vi "Beta Moments.vi"(9 "b":dbl=1.0, 10 "a":dbl=1.0) -> (0 "error":i32, 2 "variance":dbl=0.08333333333333333, 3 "mean":dbl=0.5)   [LabVIEW 2017, in "NI_Gmath.lvlib"]
doc: "Returns the expected mean and variance of the random variate X, where X describes the selected distribution type. You must manually select the polymorphic instance to use."
uses:
  <vilib>/gmath/NI_Gmath.lvlib
  <vilib>/gmath/statdist.llb/st_error_code.ctl
panel:
  # "Beta Moments"
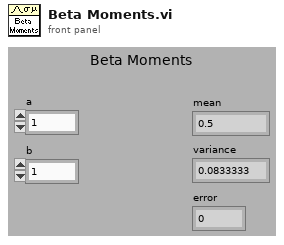
[diagram p1: front panel]
types:
  T1 = typedef "NI_Gmath.lvlib/st_error_code.ctl" = i32
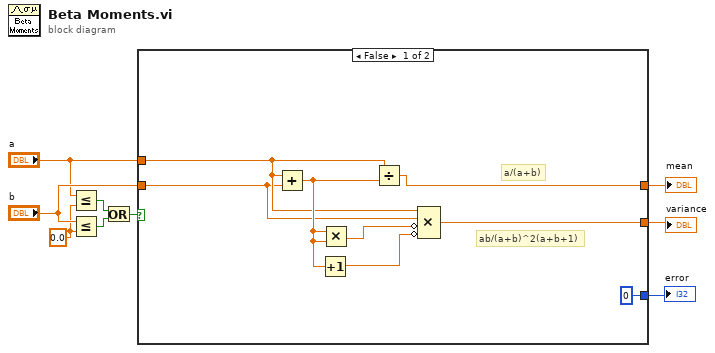
[diagram p0: block diagram]
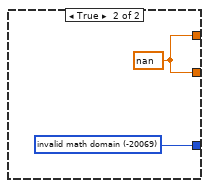
[diagram p2: hidden frame]
diagram:
  w6 = 0.0 ("y")
  n1 = Less Or Equal?(x="a", y=w6) -> (x <= y?=w2:bool)
  n2 = Less Or Equal?(x="b", y=w6) -> (x <= y?=w3:bool)
  n3 = Or(x=w2, y=w3) -> (x .or. y?=w4:bool)
  n4 = case shown="False" w4 {
    tunnel: "b" -> [w13 _]
    tunnel: [0 ("invalid math domain") w18] -> w9
    tunnel: [w16 w19] -> w8
    tunnel: "a" -> [w14 _]
    tunnel: [w10 w19] -> w1
    frame False {
      # "ab/(a+b)^2(a+b+1)"
      # "a/(a+b)"
      n5 = Add(x=w14, y=w13) -> (x+y=w15:dbl)
      n6 = Increment(x=w15) -> (x+1=w11:dbl)
      n7 = Multiply(x=w15, y=w15) -> (x*y=w12:dbl)
      n8 = Divide(x=w14, y=w15) -> (x/y=w16:dbl)
      n9 = Compound Arithmetic op=MULTIPLY(w14, w13, invert w12, invert w11) -> (w10:dbl)
    }
    frame True {
      w18 = T1 -20069 items=["invalid math domain"=-20069, "Fourier interpolation size m >= n"=-20070, "empty array"=-20003] ("stat interp error code")
      w19 = nan
    }
  }
  "mean" <- w8
  "error" <- w9
  "variance" <- w1
